vi "Sine_Scale.vi"(2 "Bypass VI function":bool, 3 "Amplify":dbl(knob)=4.036434060236755 scale=0.0..10.0, 4 "Sensor measurment\n(Degrees)":dbl, 5 "Input angle (Degrees)":dbl) -> (1 "Output":dbl)   [LabVIEW 2015]
doc: "Help by FRC Team 836 - The RoboBees\n\nThis VI produces a Sine scaled output of the input angle. The VI couples a sensor input plus an offset, both in degrees, and converts them to a Sine scaled output.\nThis Sine scaled output can be amplified before being applied to the input angle.\nThe VI also allows for a bypass function that outputs the input angle with no modifications."
panel:
  in  "Degrees of offset":dbl=67.5
  # "Maximum force on Elevator Motor\nis when linkage is at 90 deg, which is\nwhen Shooter is at 22.5 deg\n90 - 22.5 = 67.5 deg offset"
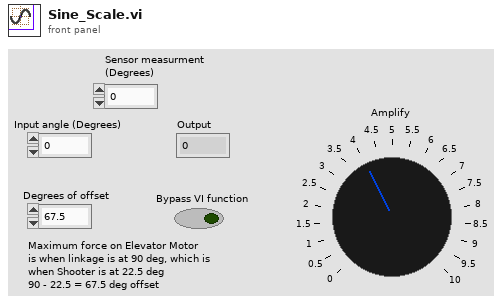
[diagram p1: front panel]
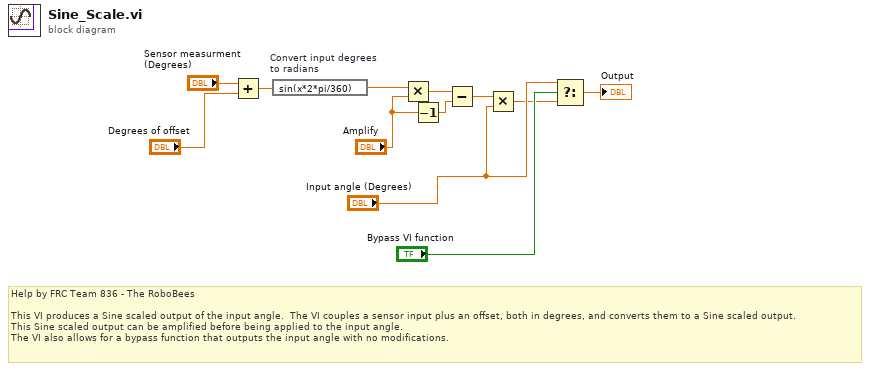
[diagram p0: block diagram]
diagram:
  # "Help by FRC Team 836 - The RoboBees\n\nThis VI produces a Sine scaled output of the input angle.  The VI couples a sensor input plus an offset, both in degrees, and converts them to a Sine scaled output.\nThis Sine scaled output can be amplified before being applied to the input angle.\nThe VI also allows for a bypass function that outputs the input angle with no modifications."
  n1 = Add(x="Sensor measurment\n(Degrees)", y="Degrees of offset") -> (x+y=w11:dbl)
  n2 = expression code="sin(x*2*pi/360)" "Convert input degrees\nto radians"(w11) -> (w10:dbl)
  n3 = Multiply(x=w10, y="Amplify") -> (x*y=w9:dbl)
  n4 = Decrement(x="Amplify") -> (x-1=w6:dbl)
  n5 = Subtract(x=w9, y=w6) -> (x-y=w7:dbl)
  n6 = Multiply(x=w7, y="Input angle (Degrees)") -> (x*y=w2:dbl)
  n7 = Select(t="Input angle (Degrees)", s="Bypass VI function", f=w2) -> (s? t:f=→"Output":dbl)
